vi "Main.vi"   [LabVIEW 2020]
uses:
  SampleCommonLib.lvlib
  SampleClass/SampleClass.lvclass
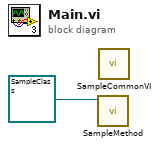
[diagram p0: block diagram]
diagram:
  n1 = call-dynamic "SampleMethod.vi"("SampleClass in"=refnum<class "SampleClass.lvclass"> refnum) -> ()  [unwired: 9 in, 2 out]
  n2 = call "SampleCommonVI.vi"() -> ()  [unwired: 12 in]
